vi "DmmPwr Triggered Measurement Example.vi"() -> ()   [LabVIEW 2017]
uses:
  DmmPwr Simulator.lvlib
panel:
  out "Measured Value":dbl
  in  "VISA resource name":refnum<visa-resource-name>="TCPIP::localhost::9997::SOCKET"
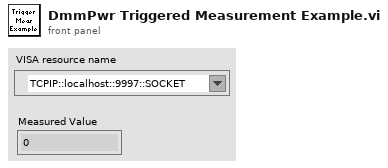
[diagram p1: front panel]
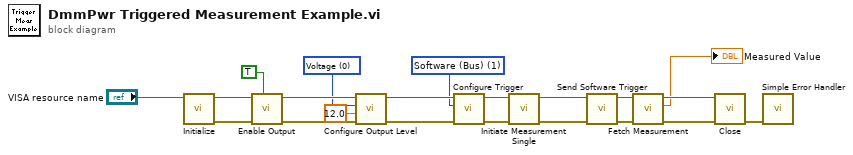
[diagram p0: block diagram]
diagram:
  w10 = 1 items=["Immediate", "Software (Bus)"] ("Trigger Source (0: Immediate)")
  w14 = u16 0 items=["Voltage", "Current"] ("Output Type (0: Voltage)")
  n1 = call "Initialize.vi"("VISA resource name"="VISA resource name") -> ("error out"=w18:errorcluster, "VISA resource name out"=w19:refnum<visa-resource-name>)  [unwired: 9 in]
  n2 = call "Enable Output.vi"("Enable Output (F: Disable)"=TRUE, "error in (no error)"=w18, "VISA resource name"=w19) -> ("error out"=w15:errorcluster, "VISA resource name out"=w16:refnum<visa-resource-name>)  [unwired: 7 in]
  n3 = call "Configure Output Level.vi"("error in (no error)"=w15, "Output Level (0)"=12.0, "Output Type (0: Voltage)"=w14, "VISA resource name"=w16) -> ("error out"=w11:errorcluster, "VISA resource name out"=w12:refnum<visa-resource-name>)  [unwired: 6 in]
  n4 = call "Configure Trigger.vi"("error in (no error)"=w11, "Trigger Source (0: Immediate)"=w10, "VISA resource name"=w12) -> ("error out"=w8:errorcluster, "VISA resource name out"=w9:refnum<visa-resource-name>)  [unwired: 7 in]
  n5 = call "Initiate Measurement Single.vi"("error in (no error)"=w8, "VISA resource name"=w9) -> ("error out"=w6:errorcluster, "VISA resource name out"=w7:refnum<visa-resource-name>)  [unwired: 8 in]
  n6 = call "Send Software Trigger.vi"("error in (no error)"=w6, "VISA resource name"=w7) -> ("error out"=w4:errorcluster, "VISA resource name out"=w5:refnum<visa-resource-name>)  [unwired: 8 in]
  n7 = call "Fetch Measurement.vi"("error in (no error)"=w4, "VISA resource name"=w5) -> ("error out"=w3:errorcluster, "Measured Value"=→"Measured Value":dbl, "VISA resource name out"=w2:refnum<visa-resource-name>)  [unwired: 7 in]
  n8 = call "Close.vi"("error in (no error)"=w3, "VISA resource name"=w2) -> ("error out"=w21:errorcluster)  [unwired: 9 in]
  n9 = call <vilib>:"Simple Error Handler.vi"("error in (no error)"=w21) -> ()  [unwired: 4 in, 5 out]
